vi "Set Side Menu Visibility.vi"(8 "error in (no error)":errorcluster, 10 "Visible":bool, 11 "UI Controller in":refnum<class "UI Controller.lvclass">) -> (0 "error out":errorcluster, 3 "UI Controller out":refnum<class "UI Controller.lvclass">)   [LabVIEW 2020, in "UI Controller.lvlib" / "UI Controller.lvclass"]
uses:
  UI Controller.lvclass
  C:/Program Files/National Instruments/LabVIEW 2020/vi.lib/ActorFrameworkMVC/View Controller/View Controller/View Controller.lvclass
  <vilib>/Utility/miscctls.llb/LVPositionTypeDef.ctl
  <vilib>/ActorFrameworkMVC/View Controller/View Controller/View Controller.lvclass
panel:
  # "NOTICE -- YOU MUST LEAVE THIS NOTICE IN PLACE.\n\nCopyright (c) 2017, LIANG LIU Shawn.Liu.cn@gmail.com\nAll rights reserved.\n\nRedistribution and use in source and binary forms, with or without modification, are permitted provided that the following conditions are met:\n-Redistributions of source code must retain the above copyright notice, this list of conditions and the following disclaimer.\n-Redistributions in binary form must reproduce the above copyright notice, this list of conditions and the following disclaimer in the documentation and/or other materials provided with the distribution.\n-Neither the name of the eLp nor the names of its contributors may be used to endorse or promote products derived from this software without specific prior written permission.\n\nTHIS SOFTWARE IS PROVIDED BY THE COPYRIGHT HOLDERS AND CONTRIBUTORS \"AS IS\" AND ANY EXPRESS OR IMPLIED WARRANTIES, INCLUDING, BUT NOT LIMITED TO, THE IMPLIED WARRANTIES OF MERCHANTABILITY AND FITNESS FOR A PARTICULAR PURPOSE ARE DISCLAIMED. IN NO EVENT SHALL THE COPYRIGHT HOLDER OR CONTRIBUTORS BE LIABLE FOR ANY DIRECT, INDIRECT, INCIDENTAL, SPECIAL, EXEMPLARY, OR CONSEQUENTIAL DAMAGES (INCLUDING, BUT NOT LIMITED TO, PROCUREMENT OF SUBSTITUTE GOODS OR SERVICES; LOSS OF USE, DATA, OR PROFITS; OR BUSINESS INTERRUPTION) HOWEVER CAUSED AND ON ANY THEORY OF LIABILITY, WHETHER IN CONTRACT, STRICT LIABILITY, OR TORT (INCLUDING NEGLIGENCE OR OTHERWISE) ARISING IN ANY WAY OUT OF THE USE OF THIS SOFTWARE, EVEN IF ADVISED OF THE POSSIBILITY OF SUCH DAMAGE."
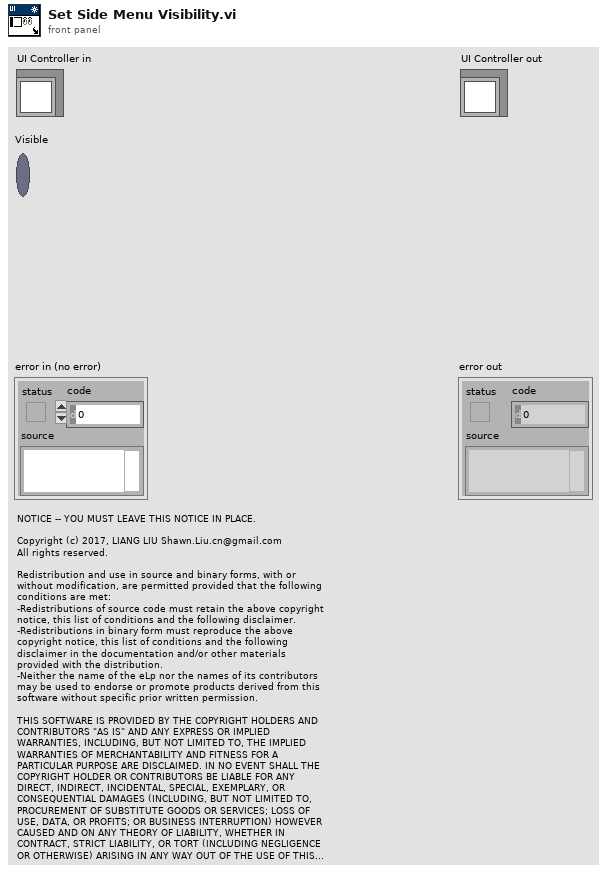
[diagram p1: front panel]
types:
  T1 = typedef "LVPositionTypeDef.ctl" = cluster{"Left":i32, "Top":i32}
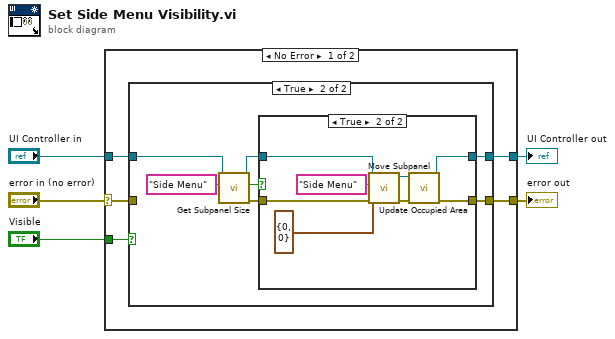
[diagram p0: block diagram]
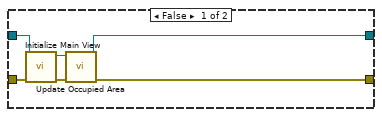
[diagram p2: hidden frame]
diagram:
  n1 = case shown="No Error" "error in (no error)" {
    selector: "error in (no error)" -> [w6 w35]
    tunnel: [w10 w35] -> w5
    tunnel: [w9 w34] -> w4
    tunnel: "UI Controller in" -> [w8 w34]
    tunnel: "Visible" -> [w7 _]
    frame No Error {
      n2 = case shown="True" w7 {
        tunnel: [w13 w23] -> w10
        tunnel: [w11 w22] -> w9
        tunnel: w8 -> [w14 w21]
        tunnel: w6 -> [w16 _]
        frame False {
          n3 = call "Initialize Main View.vi"("error in (no error)"=w16, "UI Controller in"=w14) -> ("error out"=w15:errorcluster, "UI Controller out"=w12:refnum<class "UI Controller.lvclass">)  [unwired: 8 in]
          n4 = call "Update Occupied Area.vi"("error in (no error)"=w15, "UI Controller in"=w12) -> ("error out"=w13:errorcluster, "UI Controller out"=w11:refnum<class "UI Controller.lvclass">)  [unwired: 8 in]
        }
        frame True {
          n5 = call <vilib>:"Get Subpanel Size.vi"("Subpanel Name"="Side Menu", "View Controller in"=w21) -> ("error out"=w20:errorcluster, "Found?"=w18:bool, "View Controller out"=w17:refnum<class "UI Controller.lvclass">)  [unwired: 6 in, 1 out]
          n6 = case shown="True" w18 {
            tunnel: [w25 w30] -> w23
            tunnel: [w24 w28] -> w22
            tunnel: w20 -> [w25 w29]
            tunnel: w17 -> [w24 w27]
            frame False {
            }
            frame True {
              n7 = call-dynamic "Move Subpanel.vi"("error in (no error)"=w29, "Position"=T1 {"Left"=0, "Top"=0}, "Subpanel Name"="Side Menu", "View Controller in"=w27) -> ("error out"=w32:errorcluster, "View Controller out"=w31:refnum<class "UI Controller.lvclass">)  [unwired: 6 in]
              n8 = call "Update Occupied Area.vi"("error in (no error)"=w32, "UI Controller in"=w31) -> ("error out"=w30:errorcluster, "UI Controller out"=w28:refnum<class "UI Controller.lvclass">)  [unwired: 8 in]
            }
          }
        }
      }
    }
    frame Error {
    }
  }
  "error out" <- w5
  "UI Controller out" <- w4
